vi "Get Node Data.vi"(8 "error in (no error)":errorcluster, 10 "Node Path (parent, child)":string[](array[string]), 11 "Tree Map Handle In":T3) -> (0 "error out":errorcluster, 1 "Node Exists?":bool, 2 "Node Data":T1, 3 "Tree Map Handle out":T3)   [LabVIEW 2020, in "Blue Tree Map OpenSource.lvlib"]
doc: "This will return the node data for the specified tree path"
uses:
  Blue Tree Map OpenSource.lvlib
  Typedefs/Tree Map Handle.ctl
  Typedefs/Tree Map.ctl
  Typedefs/Tree Map Data.ctl
  Typedefs/Tree Node Data.ctl
  Typedefs/Attribute Map.ctl
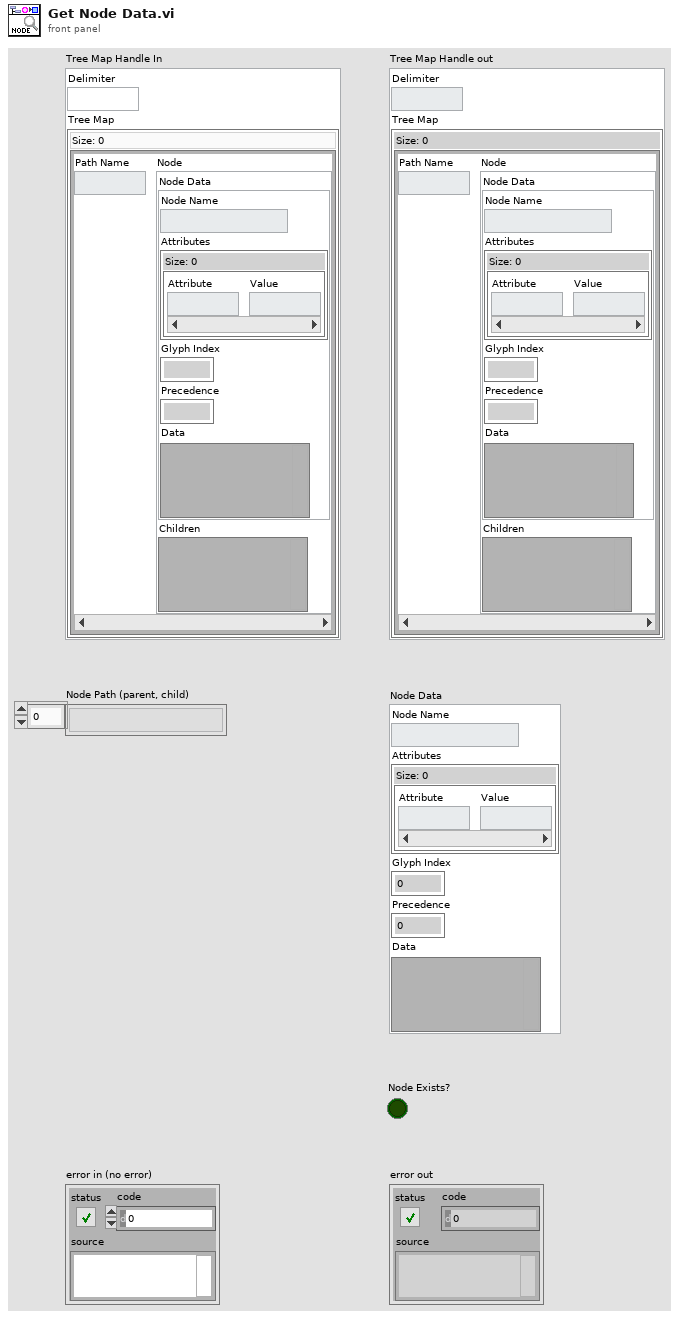
[diagram p1: front panel]
types:
  T1 = typedef "Blue Tree Map OpenSource.lvlib/Tree Node Data.ctl" = cluster{"Node Name":string, "Attributes":T2, "Glyph Index":i32, "Precedence":i32, "Data":variant}
  T2 = typedef "Blue Tree Map OpenSource.lvlib/Attribute Map.ctl" = map{string, string}
  T3 = typedef "Blue Tree Map OpenSource.lvlib/Tree Map Handle.ctl" = cluster{"Delimiter":string, "Tree Map":T4}
  T4 = typedef "Blue Tree Map OpenSource.lvlib/Tree Map.ctl" = map{string, T5}
  T5 = typedef "Blue Tree Map OpenSource.lvlib/Tree Map Data.ctl" = cluster{"Node Data":T1, "Children":variant}
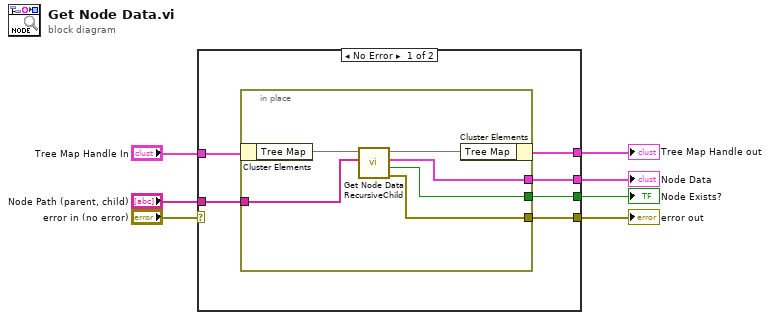
[diagram p0: block diagram]
diagram:
  n1 = case shown="No Error" "error in (no error)" {
    selector: "error in (no error)" -> [_ w21]
    tunnel: "Tree Map Handle In" -> [w13 w20]
    tunnel: "Node Path (parent, child)" -> [w12 _]
    tunnel: [w11 _] -> w5
    tunnel: [w10 w20] -> w4
    tunnel: [w9 w21] -> w3
    tunnel: [w8 _] -> w1
    frame No Error {
      n2 = in-place {
        in-place-border: w12 -> [w18]
        in-place-border: [w17] -> w8
        in-place-border: [w16] -> w11
        in-place-border: [w15] -> w9
        n3 = in-place-cluster #1(w13) -> ("Tree Map"=w19:T4)
        n4 = call "Get Node Data RecursiveChild.vi"("Node Path (parent, child)"=w18, "Tree Map In"=w19) -> ("error out"=w15:errorcluster, "Node Exists?"=w16:bool, "Node Data"=w17:T1, "Tree Map Out"=w14:T4)  [unwired: 6 in]
        n5 = in-place-cluster #1("Tree Map"=w14) -> (w10:T3)
      }
    }
    frame Error {
    }
  }
  "error out" <- w3
  "Tree Map Handle out" <- w4
  "Node Exists?" <- w5
  "Node Data" <- w1
